vi "Vent Gas.vi"(7 "Gas":string, 8 "error in (no error)":errorcluster, 11 "PAS":T1 caption="Gas") -> (0 "error out":errorcluster)   [LabVIEW 2015]
uses:
  CAN Communication/PAS/Typedefs/Session Handle.ctl
  CAN Communication/PAS/PAS.lvclass
  CAN Communication/PAS/Typedefs/Valves.ctl
  User Interface/UI Handler/UI Handler.lvclass
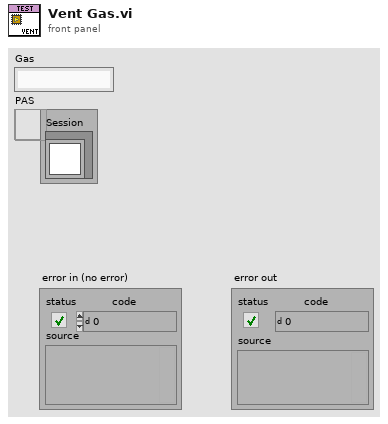
[diagram p1: front panel]
types:
  T1 = typedef "PAS.lvclass/Session Handle.ctl" = refnum<data-value>
  T2 = typedef "PAS.lvclass/Valves.ctl" = u16
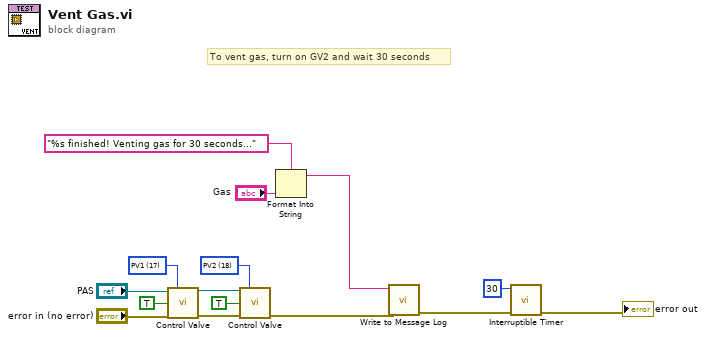
[diagram p0: block diagram]
diagram:
  w5 = T2 18 items=["PV1"=17, "PV2"=18, "PV3"=19, "PV4"=20] ("Valves")
  w6 = T2 17 items=["PV1"=17, "PV2"=18, "PV3"=19, "PV4"=20] ("Valves")
  # "To vent gas, turn on GV2 and wait 30 seconds"
  n1 = call "Control Valve.vi"("Session Handle in"="PAS", "Valves"=w6, "Energize?"=TRUE, "error in (no error)"="error in (no error)") -> ("Session Handle out"=w3:T1, "error out"=w2:errorcluster)  [unwired: 8 in, 2 out]
  n2 = call "Control Valve.vi"("Session Handle in"=w3, "Valves"=w5, "Energize?"=TRUE, "error in (no error)"=w2) -> ("error out"=w1:errorcluster)  [unwired: 8 in, 3 out]
  n3 = Format Into String(format string="%s finished! Venting gas for 30 seconds...", "Gas") -> (resulting string=w11:string)  [unwired: 2 in, 1 out]
  n4 = call "Write to Message Log.vi"("error in (no error)"=w1, "Message"=w11) -> ("error out"=w14:errorcluster)  [unwired: 9 in]
  n5 = call "Interruptible Timer.vi"("error in (no error)"=w14, "Wait (s)"=30) -> ("error out"=→"error out":errorcluster)  [unwired: 7 in, 2 out]
